vi "Read Timing.vi"(8 "error in (no error)":errorcluster, 11 "Display Console in":refnum<class "Display Console.lvclass">) -> (0 "error out":errorcluster, 2 "timing":dbl, 3 "Display Console out":refnum<class "Display Console.lvclass">)   [LabVIEW 2019, in "Display Console Actor.lvlib" / "Display Console.lvclass"]
uses:
  Display Console.lvclass
  Abstract Display Console Actor/Abstract Display Console Actor/Abstract Display Console.lvclass
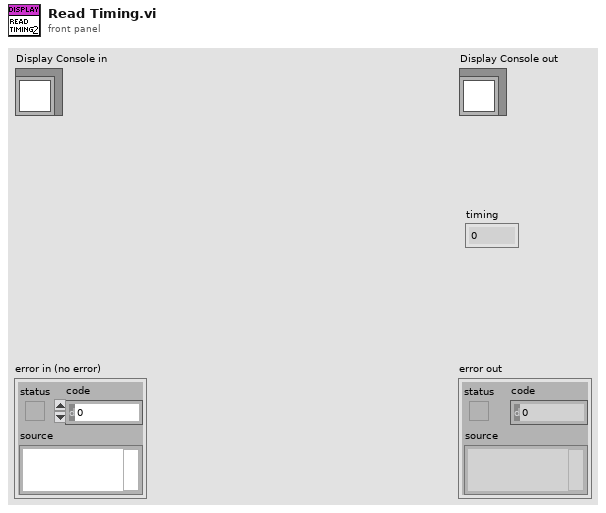
[diagram p1: front panel]
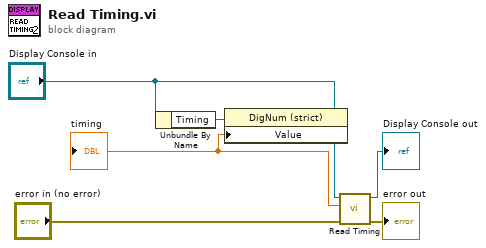
[diagram p0: block diagram]
diagram:
  n1 = Unbundle By Name("Display Console in") -> ("Timing"=w3:refnum<vi>)
  n2 = property class="DigNum (strict)"(reference=w3, "Value"="timing") -> ()  [unwired: 1 in, 2 out]
  n3 = call-parent "Read Timing.vi"("error in (no error)"="error in (no error)", 10:"timing", "Abstract Display Console in"="Display Console in") -> ("error out"=→"error out":errorcluster, "Abstract Display Console out"=→"Display Console out":refnum<class "Display Console.lvclass">)  [unwired: 6 in, 1 out]
